vi "action - BuildSystem.vi"(8 "error in (no error)":errorcluster, 11 "Path":path) -> (3 "f":string)   [LabVIEW 2019]
uses:
  <vilib>/AppBuilder/AB_API_Simple/Build (path).vi
  <vilib>/AppBuilder/AB_API_Simple/NI_App_Builder_API.lvlib
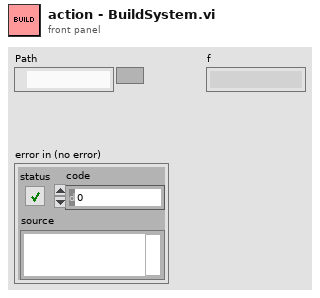
[diagram p1: front panel]
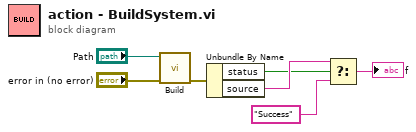
[diagram p0: block diagram]
diagram:
  n1 = call-poly <vilib>:"Build.vi"("error in (no error)"="error in (no error)", "Path to project"="Path") -> ("error out"=w6:errorcluster)  [unwired: 8 in, 1 out]
  n2 = Unbundle By Name(w6) -> ("status"=w1:bool, "source"=w2:string)
  n3 = Select(t=w2, s=w1, f="Success") -> (s? t:f=→"f":string)
